vi "close.vi"(8 "error in (no error)":errorcluster, 11 "NetworkPixelfly in":refnum<class "NetworkPixelfly.lvclass">) -> (0 "error out":errorcluster)   [LabVIEW 2011, in "Hardware.lvlib" / "HWControllers.lvlib" / "NetworkPixelfly.lvclass"]
uses:
  NetworkPixelfly.lvclass
  NetworkPixelfly.lvclass/NetworkPixelfly.ctl
  Channels/Camera/PixelflySA/PixelflySA.lvclass
  NetworkCamera.lvclass
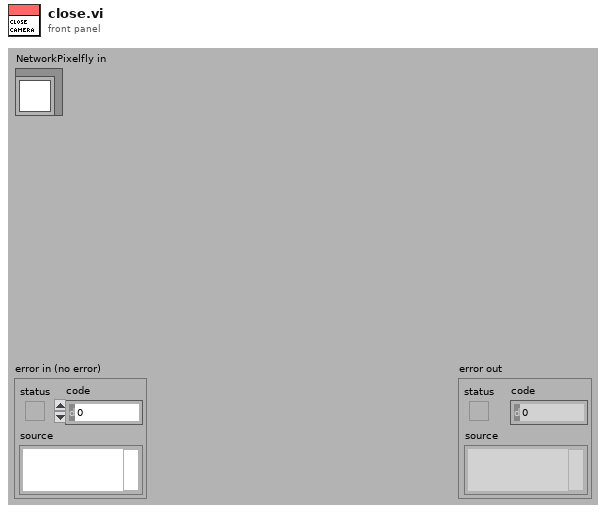
[diagram p1: front panel]
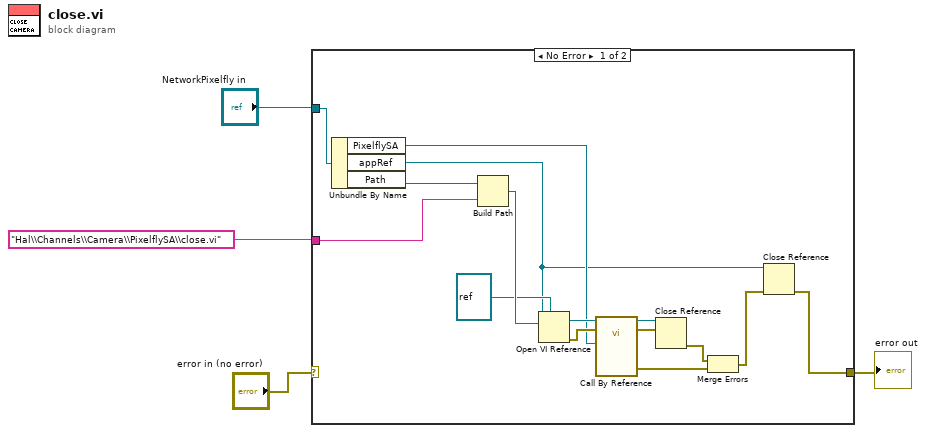
[diagram p0: block diagram]
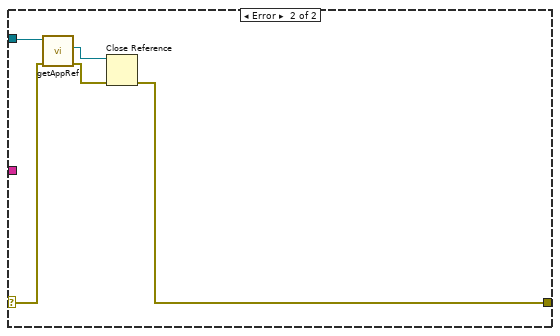
[diagram p2: hidden frame]
diagram:
  n1 = case shown="No Error" "error in (no error)" {
    selector: "error in (no error)" -> [_ w23]
    tunnel: [w16 w20] -> w1
    tunnel: "NetworkPixelfly in" -> [w15 w24]
    tunnel: "Hal\\Channels\\Camera\\PixelflySA\\close.vi" ("viPath") -> [w18 _]
    frame No Error {
      n2 = Unbundle By Name(w15) -> ("PixelflySA"=w10:refnum<class "PixelflySA.lvclass">, "appRef"=w5:refnum<vi>, "Path"=w14:path)
      n3 = Build Path(base path=w14, name or relative path=w18) -> (appended path=w19:path)
      n4 = Open VI Reference(type specifier VI Refnum (for type only)=refnum<vi> refnum, application reference (local)=w5, vi path=w19) -> (vi reference=w11:refnum<vi>, error out=w12:errorcluster)  [unwired: 3 in]
      n5 = call-by-ref "?"(reference=w11, error in=w12, "Pixelfly in"=w10) -> (reference out=w8:refnum<vi>, error out=w9:errorcluster, 0:"error out"=w6:errorcluster)  [unwired: 10 in]
      n6 = Close Reference(reference=w8, error in (no error)=w9) -> (error out=w7:errorcluster)
      n7 = Merge Errors(w7, w6) -> (w17:errorcluster)
      n8 = Close Reference(reference=w5, error in (no error)=w17) -> (error out=w16:errorcluster)
    }
    frame Error {
      n9 = call "getAppRef.vi"("error in (no error)"=w23, "NetworkCamera in"=w24) -> ("error out"=w21:errorcluster, "appRef"=w22:refnum<vi>)  [unwired: 7 in, 1 out]
      n10 = Close Reference(reference=w22, error in (no error)=w21) -> (error out=w20:errorcluster)
    }
  }
  "error out" <- w1
